vi "PH_Beckhoff-16BB.ProcPeriodic.vi"(0 "i ref in":refnum<vi>, 3 "ms timeout (10000)":i32=10000, 5 "error in (no error)":errorcluster) -> (14 "i ref out":refnum<vi>, 17 "timed out":bool, 19 "error out":errorcluster)   [LabVIEW 2014, in "PH_Beckhoff-16BB.lvlib"]
doc: "This method serves to periodically do things like reading values from the HW. Methods that should be executed periodically should be called from THIS methode. Add code here."
uses:
  PH_Beckhoff-16BB.lvlib
  PH_Beckhoff/PH_Beckhoff.lvlib
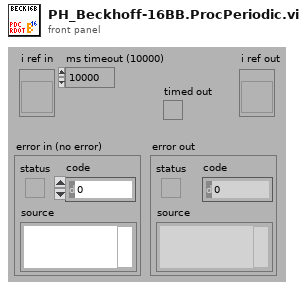
[diagram p1: front panel]
types:
  T1 = typedef "PH_Beckhoff-16BB.lvlib/PH_Beckhoff-16BB.i attribute.ctl" = cluster{"PA Chiller":cluster{"PSDB":cluster{"Status Service ID":i32, "Instance ID":i32, "Data Status":T2, "Ref Status":refnum<vi>, "Error Code":i32}, "Status":cluster{"GUI Ref":refnum<vi>, "Status Service ID":i32, "Status":T3}, "DIs":cluster{"Flow Control":cluster{"GUI Ref":refnum<vi>, "# in Data":i32}, "High-Temp":cluster{"GUI Ref":refnum<vi>, "# in Data":i32}, "Conductivity":cluster{"GUI Ref":refnum<vi>, "# in Data":i32}, "Niveau":cluster{"GUI Ref":refnum<vi>, "# in Data":i32}}, "PSDB Thread":cluster{"Ref":refnum<vi>, "Q-Ref":refnum<queue>}}, "PSDB":cluster{"Shot #":i32, "Subsystem":T4}, "Racktype":string, "PSDB Credentials":T5}
  T2 = typedef "PH_PSDBWriter.lvlib/PH_PSDBWriter.Data Status.ctl" = i16
  T3 = typedef "PH_StatusHandler.lvlib/PH_StatusHandler.Status.ctl" = i16
  T4 = typedef "PH_PSDBWriter.lvlib/PH_PSDBWriter.PHELIX-Subsystems.ctl" = i32
  T5 = typedef "PH_Common.lvlib/PH_Connection.PSDB Credentials.ctl" = cluster{"PW":string, "ID":string, "DS":string}
  T6 = typedef "PH_Beckhoff.lvlib/PH_Beckhoff.i attribute.ctl" = cluster{"GUI Refs":T7, "operation?":bool, "Default Prdc Interval":i32, "Connection":T8, "AMS Net ID":T9, "Klemmencluster: # of":T10, "Values":T11, "IP":string, "Description":string, "configured?":bool, "Change Manager":cluster{"Detemination wanted?":bool, "Values changed at":cluster{"Sonderklemmen Inputs":i32[], "Analog Inputs":i32[], "Analog Outputs":i32[], "Digital Inputs":i32[], "Digital Outputs":i32[]}}, "Difference to handle an analog input as change":u32}
  T7 = typedef "PH_Beckhoff.lvlib/PH_Beckhoff.GUI Refs.ctl" = cluster{"ADS Error":refnum<vi>, "Values":refnum<vi>, "configured?":refnum<vi>, "Connection":refnum<vi>, "IP":refnum<vi>, "Prdc Int [ms]":refnum<vi>}
  T8 = typedef "PH_Beckhoff.lvlib/PH_Beckhoff.Connectivity.ctl" = cluster{"DLL?":bool, "Port?":bool, "Client?":bool, "Ping?":bool, "unsuccessful Pings":u32}
  T9 = typedef "Beckhoff - Driver np.lvlib/Beckhoff Access.ctl" = cluster{"DLL path":path, "AMS Net ID":cluster{"1st # of IP":u8, "2nd # of IP":u8, "3rd # of IP":u8, "4th # of IP":u8, "In Port":u8, "Out Port":u8}}
  T10 = typedef "Beckhoff - Driver np.lvlib/Klemmendeclarer.ctl" = cluster{"Offset due to Sonderklemms":u32, "analog Inputs":u32, "analog Outputs":u32, "digital Input Bits":u32, "digital Output Bits":u32}
  T11 = typedef "PH_Beckhoff.lvlib/PH_Beckhoff.Values.ctl" = cluster{"Sonderklemmen Inputs":T12, "Analog Inputs":T13, "Analog Outputs":T15, "Digital Inputs":T16, "Digital Outputs":T17}
  T12 = typedef "PH_Beckhoff.lvlib/PH_Beckhoff.Sonderklemmen Inputs.ctl" = cluster{"Total Length":u32, "Name":string, "Value":u64, "Quality":bool, "Service ID":i32, "Offset":u32, "Length":u32}[]
  T13 = typedef "PH_Beckhoff.lvlib/PH_Beckhoff.Analog Inputs.ctl" = cluster{"Name":string, "Value":u32, "Quality":bool, "Service ID":i32, "Sca Type":T14}[]
  T14 = typedef "PH_Beckhoff.lvlib/PH_Beckhoff.Scaling Type.ctl" = enum16{"none", "0 ... 15 Bit -> 0 ... 5", "0 ... 15 Bit -> 0 ... 10", "0 ... 15 Bit -> 0 ... 25", "0 ... 15 Bit -> 4 ... 20", "0 ... 15 Bit -> 0 ... 1", "0 ... 15 Bit -> 0 ... 20000", "0 ... 15 Bit -> 0 ... 24000"}
  T15 = typedef "PH_Beckhoff.lvlib/PH_Beckhoff.Analog Outputs.ctl" = cluster{"Name":string, "Value":u32, "Quality":bool, "Wanted Value":u32, "Service ID":i32, "Sca Type":T14}[]
  T16 = typedef "PH_Beckhoff.lvlib/PH_Beckhoff.Digital Inputs.ctl" = cluster{"Name":string, "Value":bool, "Quality":bool, "Service ID":i32, "inverted?":bool}[]
  T17 = typedef "PH_Beckhoff.lvlib/PH_Beckhoff.Digital Outputs.ctl" = cluster{"Name":string, "Value":bool, "Quality":bool, "Wanted Value":bool, "Service ID":i32, "inverted?":bool}[]
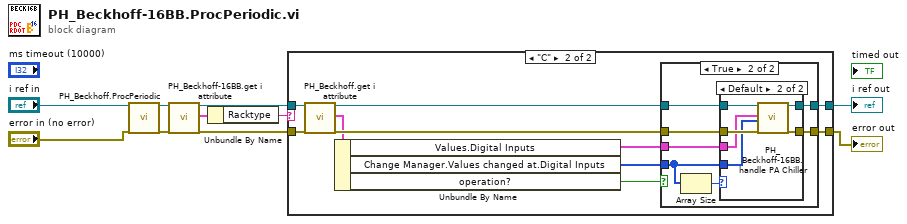
[diagram p0: block diagram]
diagram:
  n1 = call "PH_Beckhoff.ProcPeriodic.vi"("i ref in"="i ref in", "error in (no error)"="error in (no error)") -> ("i ref out"=w7:refnum<vi>, "error out"=w8:errorcluster)  [unwired: 15 in, 1 out]
  n2 = call "PH_Beckhoff-16BB.get i attribute.vi"("i ref in"=w7, "error in (no error)"=w8) -> ("i ref out"=w6:refnum<vi>, "i attribute"=w2:T1, "error out"=w4:errorcluster)  [unwired: 15 in]
  n3 = Unbundle By Name(w2) -> ("Racktype"=w1:string)
  n4 = case shown="\"C\"" w1 {
    tunnel: w6 -> [w12 w18]
    tunnel: [w12 w21] -> w5
    tunnel: w4 -> [w11 w22]
    tunnel: [w11 w15] -> w3
    frame Default {
    }
    frame "C" {
      n5 = call "PH_Beckhoff.get i attribute.vi"("i ref in"=w18, "error in (no error)"=w22) -> ("i ref out"=w17:refnum<vi>, "i attribute"=w19:T6, "error out"=w20:errorcluster)  [unwired: 15 in]
      n6 = Unbundle By Name(w19) -> ("Values.Digital Inputs"=w16:T16, "Change Manager.Values changed at.Digital Inputs"=w14:i32[], "operation?"=w13:bool)
      n7 = case shown="True" w13 {
        tunnel: [w24 w31] -> w21
        tunnel: w20 -> [w23 w30]
        tunnel: w17 -> [w24 w29]
        tunnel: w16 -> [_ w28]
        tunnel: [w23 w27] -> w15
        tunnel: w14 -> [_ w25]
        frame False {
        }
        frame True {
          n8 = Array Size(array=w25) -> (size(s)=w26:i32)
          n9 = case shown="Default" w26 {
            tunnel: [w33 w38] -> w31
            tunnel: w30 -> [w32 w37]
            tunnel: w29 -> [w33 w39]
            tunnel: w28 -> [_ w35]
            tunnel: [w32 w36] -> w27
            tunnel: w25 -> [_ w34]
            frame 0 {
            }
            frame Default {
              n10 = call "PH_Beckhoff-16BB.handle PA Chiller.vi"("i ref in"=w39, "Current Digital Inputs"=w35, "changed DE Values"=w34, "error in"=w37) -> ("i ref out"=w38:refnum<vi>, "error out"=w36:errorcluster)  [unwired: 14 in]
            }
          }
        }
      }
    }
  }
  "error out" <- w3
  "i ref out" <- w5
